vi "zad1.vi"() -> ()   [LabVIEW 2018]
uses:
  LVMQTT-master/LVMQTT-master/Controls/QoS.ctl
  LVMQTT-master/LVMQTT-master/Controls/DUP_Flag.ctl
  LVMQTT-master/LVMQTT-master/Controls/Retain_Flag.ctl
  LVMQTT-master/LVMQTT-master/Controls/Connect_Flags.ctl
  LVMQTT-master/LVMQTT-master/Controls/Will_Info.ctl
  LVMQTT-master/LVMQTT-master/Controls/User_Info.ctl
  LVMQTT-master/LVMQTT-master/Controls/Connection_Return_Codes.ctl
  LVMQTT-master/LVMQTT-master/Controls/MessageType.ctl
  LVMQTT-master/LVMQTT-master/MQTT_Functions.lvlib
panel:
  in  "stop":bool
  in  "Subscription Info Array":cluster{"Topic":string, "QoS":T1}[](array[cluster])=[{"Topic"="a/b", "QoS"=enum."At least once"}]
  out "Connection Status":T2=enum."Connection refused: not authorized"
  in  "MQTT Broker":cluster{"address (IP)":string, "port":u16}={"address (IP)"="broker.mqttdashboard.com", "port"=1883}
  in  "User Info":T3={"User Name"="User", "Password"="password"}
  in  "Will Info":T4={"Will message"="Last Will", "Will Topic"="Will Topic"}
  in  "Client ID":string="LabVIEW_MQTT_Client"
  in  "Connect Flags":T5
  in  "Connect Meta":T8={"QoS"=enum."At most once", "DUP"=FALSE, "Retain"=TRUE, "Keep Alive (sec)"=60}
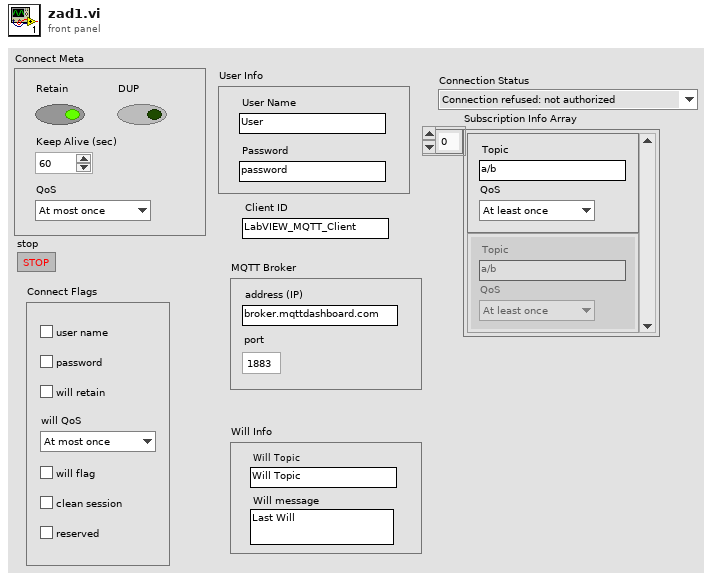
[diagram p1: front panel]
types:
  T1 = typedef "MQTT_Functions.lvlib/QoS.ctl" = enum8{"At most once", "At least once", "Exactly once", "Reserved"}
  T2 = typedef "MQTT_Functions.lvlib/Connection_Return_Codes.ctl" = enum16{"Connection accepted", "Connection refused: unacceptable protocol version", "Connection refused: identifier rejected", "Connection refused: Server unavailable", "Connection refused: bad user name or password", "Connection refused: not authorized"}
  T3 = typedef "MQTT_Functions.lvlib/User_Info.ctl" = cluster{"User Name":string, "Password":string}
  T4 = typedef "MQTT_Functions.lvlib/Will_Info.ctl" = cluster{"Will message":string, "Will Topic":string}
  T5 = typedef "MQTT_Functions.lvlib/Connect_Flags.ctl" = cluster{"user name":bool, "password":bool, "will retain":bool, "will flag":bool, "clean session":bool, "reserved":bool, "will QoS":T1}
  T6 = typedef "MQTT_Functions.lvlib/DUP_Flag.ctl" = bool
  T7 = typedef "MQTT_Functions.lvlib/Retain_Flag.ctl" = bool
  T8 = cluster{"QoS":T1, "DUP":T6, "Retain":T7, "Keep Alive (sec)":u16}
  T9 = typedef "MQTT_Functions.lvlib/MessageType.ctl" = enum32{"Reserved", "CONNECT", "CONNACK", "PUBLISH", "PUBACK", "PUBREC", "PUBREL", "PUBCOMP", "SUBSCRIBE", "SUBACK", "UNSUBSCRIBE", "UNSUBACK", "PINGREQ", "PINGRESP", "DISCONNECT", "Reserved2"}
  T10 = cluster{"Topic Name":string, "Message":string, "Message ID":u16, "MessageType":T9}[]
  T11 = cluster{"Topic Name":string, "Message":string, "Message ID":u16, "MessageType":T9}
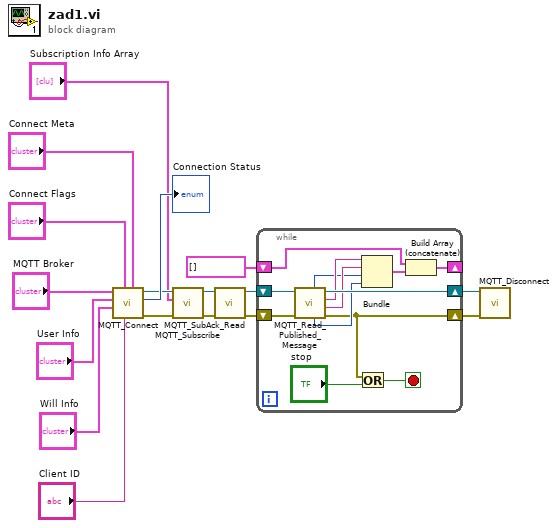
[diagram p0: block diagram]
diagram:
  n1 = call "MQTT_Connect.vi"("Connect Meta"="Connect Meta", "Client ID"="Client ID", "Connect Flags"="Connect Flags", "Will Info"="Will Info", "User Info"="User Info", "MQTT Broker"="MQTT Broker") -> ("error out"=w8:errorcluster, "Connection Status"=→"Connection Status":T2, "connection ID out"=w10:refnum<k5>)  [unwired: 3 in]
  n2 = call "MQTT_Subscribe.vi"("error in (no error)"=w8, "Subscription Info Array"="Subscription Info Array", "connection ID"=w10) -> ("error out"=w3:errorcluster, "connection ID out"=w5:refnum<k5>)  [unwired: 7 in]
  n3 = call "MQTT_SubAck_Read.vi"("error in (no error)"=w3, "connection ID"=w5) -> ("error out"=w2:errorcluster, "connection ID out"=w4:refnum<k5>)  [unwired: 7 in, 1 out]
  n4 = while {
    shift-right: [w30] -> w7
    shift-left: w4 -> [w29]
    shift-right: [w20] -> w6
    shift-left: w2 -> [w28]
    shift-right: [w22] -> _
    shift-left: T10 [] -> [w21]
    stop <- w18 stop-if-true
    n5 = call "MQTT_Read_Published_Message.vi"("error in (no error)"=w28, "connection ID"=w29) -> ("error out"=w20:errorcluster, "Message"=w26:string, "Topic Name"=w27:string, "connection ID out"=w30:refnum<k5>, "MessageType"=w24:T9, "Message ID"=w25:u16)  [unwired: 4 in]
    n6 = Or(x=w20, y="stop") -> (x .or. y?=w18:bool)
    n7 = Bundle("Topic Name"=w27, "Message"=w26, "Message ID"=w25, "MessageType"=w24) -> (w23:T11)  [unwired: 1 in]
    n8 = Build Array (concatenate)(w21, w23) -> (w22:T10)
  }
  n9 = call "MQTT_Disconnect.vi"("error in (no error)"=w6, "connection ID"=w7) -> ()  [unwired: 9 in, 1 out]
